vi "XBee example.vi"() -> ()   [LabVIEW 2012]
panel:
  out "IR array":cluster{i32, i32, i16[]}(graph)
  out "IR Index":i32
  out "Dist":i16
  out "Desired \nVelocity":i16=5
  out "Local\nHeading":i16=90
  out "Mode":i16=1
  out "Battery\nVolts":i16
  out "error out":errorcluster
  in  "error in":errorcluster
  in  "VISA resource name":refnum<visa-resource-name>="COM10"
  out "String Received":string
  out "String":string="$B^"
  in  "stop":bool caption="ESTOP"
  out "return count":u32
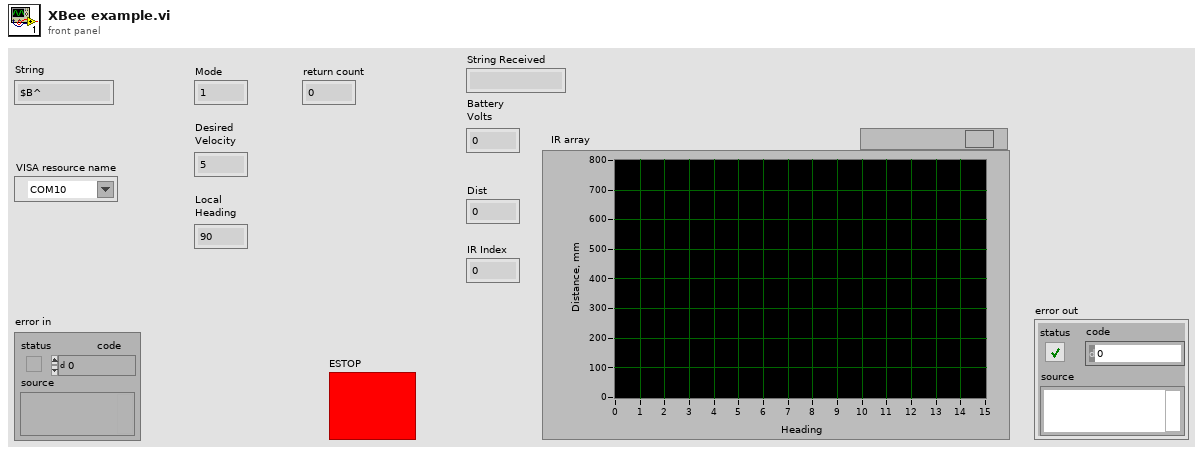
[diagram p1: front panel]
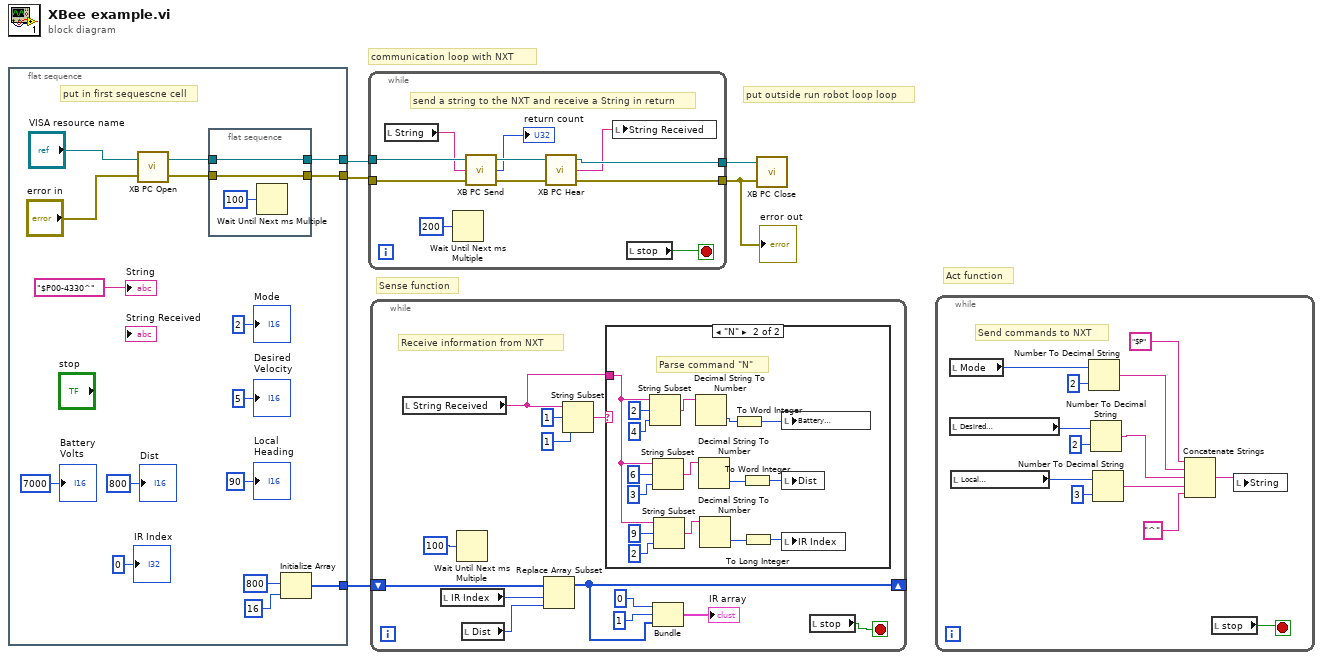
[diagram p0: block diagram]
diagram:
  # "put outside run robot loop loop"
  # "Act function"
  # "Sense function"
  # "communication loop with NXT"
  n1 = flat-sequence {
    tunnel: [w17] -> w3
    tunnel: [w16] -> w2
    tunnel: [w6] -> w1
    frame #0 {
      # "put in first sequescne cell"
      n2 = call "XB PC Open.vi"("error in (no error)"="error in", "VISA resource name"="VISA resource name") -> ("error out"=w20:errorcluster, "VISA resource name out"=w21:refnum<visa-resource-name>)
      n3 = flat-sequence {
        tunnel: w21 -> [w22]
        tunnel: w20 -> [w23]
        tunnel: [w23] -> w16
        tunnel: [w22] -> w17
        frame #0 {
          n4 = Wait Until Next ms Multiple(millisecond multiple=u32 100) -> ()  [unwired: 1 out]
        }
      }
      n5 = Initialize Array(i16 800, 16 ("dimension size")) -> (w6:i16[])
      "String" <- "$P00-4330^"
      "Battery\nVolts" <- i16 7000 ("Battery\nVolts")
      "Mode" <- i16 2 ("Mode")
      "Local\nHeading" <- i16 90 ("Local\nHeading")
      "Desired \nVelocity" <- i16 5 ("Desired \nVelocity")
      "Dist" <- i16 800 ("Dist")
      "IR Index" <- 0 ("IR Index")
    }
  }
  n6 = while {
    tunnel: w3 -> [w35]
    tunnel: w2 -> [w34]
    tunnel: [w31] -> w4
    tunnel: [w30] -> w5
    stop <- w29 stop-if-true
    # "send a string to the NXT and receive a String in return"
    n7 = local read "String"() -> (w27:string)
    n8 = Wait Until Next ms Multiple(millisecond multiple=u32 200) -> ()  [unwired: 1 out]
    n9 = call "XB PC Send.vi"("error in (no error)"=w34, "String"=w27, "VISA resource name"=w35) -> ("error out"=w33:errorcluster, "return count"=→"return count":u32, "VISA resource name out"=w32:refnum<visa-resource-name>)
    n10 = call "XB PC Hear.vi"("VISA resource name"=w32, "error in (no error)"=w33) -> ("VISA resource name out"=w30:refnum<visa-resource-name>, "String Received"=w26:string, "error out"=w31:errorcluster)
    n11 = local write "String Received"(w26) -> ()
    n12 = local read "stop"() -> (w29:bool)
  }
  "error out" <- w4
  n13 = while {
    shift-right: [w37] -> _
    shift-left: w1 -> [w42]
    stop <- w43 stop-if-true
    # "Receive information from NXT"
    n14 = local read "String Received"() -> (w48:string)
    n15 = local read "IR Index"() -> (w41:i32)
    n16 = Wait Until Next ms Multiple(millisecond multiple=u32 100) -> ()  [unwired: 1 out]
    n17 = local read "Dist"() -> (w40:i16)
    n18 = Replace Array Subset(array=w42, new element=w40, index=w41) -> (w37:i16[])
    n19 = String Subset(string=w48, offset (0)=1, length (rest)=1 ("length (rest)")) -> (substring=w47:string)
    n20 = case shown="\"N\"" w47 {
      tunnel: w48 -> [_ w50]
      frame Default {
      }
      frame "N" {
        # "Parse command \"N\""
        n21 = String Subset(string=w50, offset (0)=2, length (rest)=4 ("length (rest)")) -> (substring=w61:string)
        n22 = String Subset(string=w50, offset (0)=6, length (rest)=3 ("length (rest)")) -> (substring=w57:string)
        n23 = String Subset(string=w50, offset (0)=9, length (rest)=2 ("length (rest)")) -> (substring=w53:string)
        n24 = Decimal String To Number(string=w61) -> (number=w64:i32)  [unwired: 2 in, 1 out]
        n25 = Decimal String To Number(string=w57) -> (number=w56:i32)  [unwired: 2 in, 1 out]
        n26 = Decimal String To Number(string=w53) -> (number=w54:i32)  [unwired: 2 in, 1 out]
        n27 = To Word Integer(number=w64) -> (16bit integer=w60:i16)
        n28 = To Word Integer(number=w56) -> (16bit integer=w55:i16)
        n29 = To Long Integer(number=w54) -> (32bit integer=w49:i32)
        n30 = local write "Battery\nVolts"(w60) -> ()
        n31 = local write "Dist"(w55) -> ()
        n32 = local write "IR Index"(w49) -> ()
      }
    }
    n33 = Bundle(0, 1, w37) -> (→"IR array":cluster{i32, i32, i16[]})  [unwired: 1 in]
    n34 = local read "stop"() -> (w43:bool)
  }
  n35 = call "XB PC Close.vi"("error in (no error)"=w4, "VISA resource name"=w5) -> ()
  n36 = while {
    stop <- w66 stop-if-true
    # "Send commands to NXT"
    n37 = local read "Mode"() -> (w67:i16)
    n38 = local read "Desired \nVelocity"() -> (w68:i16)
    n39 = local read "Local\nHeading"() -> (w69:i16)
    n40 = Number To Decimal String(number=w67, width (-)=i16 2) -> (decimal integer string=w73:string)
    n41 = Number To Decimal String(number=w68, width (-)=i16 2) -> (decimal integer string=w72:string)
    n42 = Number To Decimal String(number=w69, width (-)=i16 3) -> (decimal integer string=w71:string)
    n43 = Concatenate Strings("$P", w73, w72, w71, "^") -> (w70:string)
    n44 = local read "stop"() -> (w66:bool)
    n45 = local write "String"(w70) -> ()
  }
